vi "LeCroy.Trigger Set to Normal Mode.vi"(8 "Error In":errorcluster, 11 "LeCroy.Session in":T1) -> (0 "Error Out":errorcluster, 3 "LeCroy.Session out":T1)   [LabVIEW 2018]
uses:
  typedefs/LeCroy.Session.ctl
  Driver/lecroy_wave_series/LeCroy Wave Series/LeCroy Wave Series.lvlib
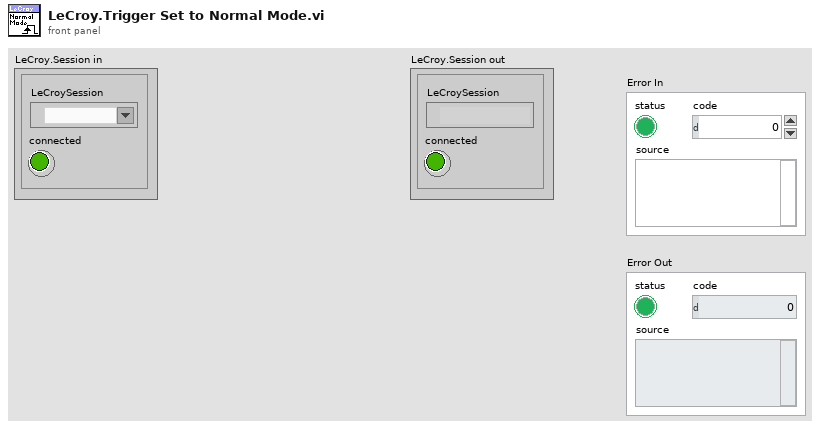
[diagram p1: front panel]
types:
  T1 = typedef "LeCroy.Session.ctl" = cluster{"LeCroySession":refnum<visa-resource-name>, "connected":bool}
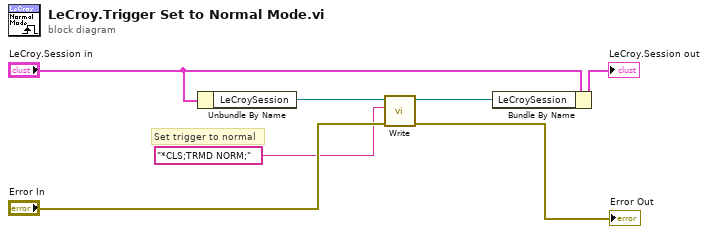
[diagram p0: block diagram]
diagram:
  # "Set trigger to normal"
  n1 = Unbundle By Name("LeCroy.Session in") -> ("LeCroySession"=w3:refnum<visa-resource-name>)
  n2 = call "Write.vi"("error in (no error)"="Error In", "Write Buffer"="*CLS;TRMD NORM;" ("Initiate"), "VISA resource name"=w3) -> ("error out"=→"Error Out":errorcluster, "VISA resource name out"=w5:refnum<visa-resource-name>)  [unwired: 7 in]
  n3 = Bundle By Name(cluster="LeCroy.Session in", "LeCroySession"=w5) -> (→"LeCroy.Session out":T1)
